vi "Initialize KUKA youBot Arm.vi"(8 "error in (no error)":errorcluster, 11 "KUKA youBot arm in":refnum<class "NI_Robotics_KUKA youBot Arm.lvclass">) -> (0 "error out":errorcluster, 3 "KUKA youBot arm out":refnum<class "NI_Robotics_KUKA youBot Arm.lvclass">)   [LabVIEW 2017, in "NI_Robotics_KUKA youBot Host.lvlib" / "NI_Robotics_KUKA youBot Arm.lvclass"]
uses:
  <vilib>/robotics/KUKA youBot/Basic Device/Arm/NI_Robotics_KUKA youBot Arm.lvclass
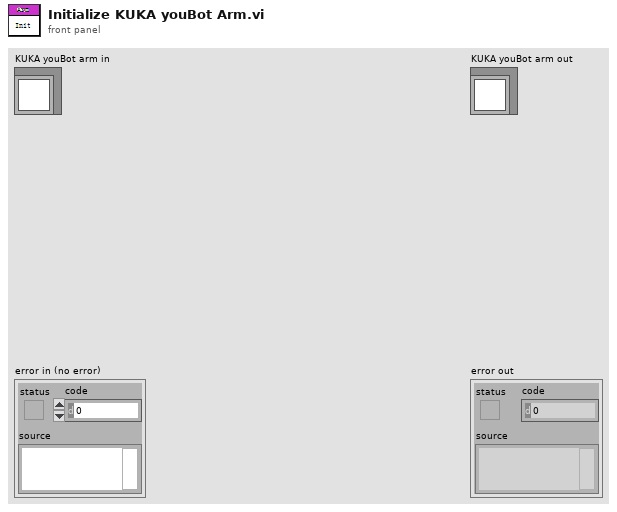
[diagram p1: front panel]
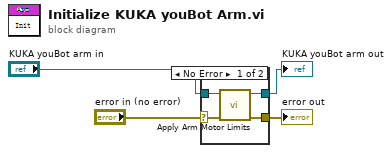
[diagram p0: block diagram]
diagram:
  n1 = case shown="No Error" "error in (no error)" {
    selector: "error in (no error)" -> [w6 w9]
    tunnel: "KUKA youBot arm in" -> [w8 w10]
    tunnel: [w7 w10] -> w2
    tunnel: [w5 w9] -> w1
    frame No Error {
      n2 = call <vilib>:"Apply Arm Motor Limits.vi"("error in (no error)"=w6, "KUKA youBot arm in"=w8) -> ("error out"=w5:errorcluster, "KUKA youBot arm out"=w7:refnum<class "NI_Robotics_KUKA youBot Arm.lvclass">)  [unwired: 8 in]
    }
    frame Error {
    }
  }
  "error out" <- w1
  "KUKA youBot arm out" <- w2
